vi "Send selected product.vi"(8 "error in (no error)":errorcluster, 10 "Product":i32, 11 "Coffee Actor in":refnum<class "Coffee Actor.lvclass">) -> (0 "error out":errorcluster, 3 "Coffee Actor out":refnum<class "Coffee Actor.lvclass">)   [LabVIEW 2020]
uses:
  <vilib>/ActorFramework/Actor/Actor.lvclass
  UI Actor Messages/Product Selected Msg/Product Selected Msg.lvclass
  Coffee Actor.lvclass
  C:/Program Files/National Instruments/LabVIEW 2020/vi.lib/ActorFramework/Actor/Actor.lvclass
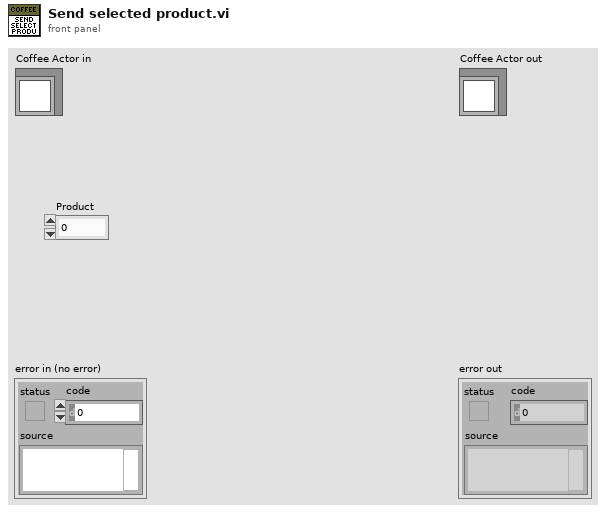
[diagram p1: front panel]
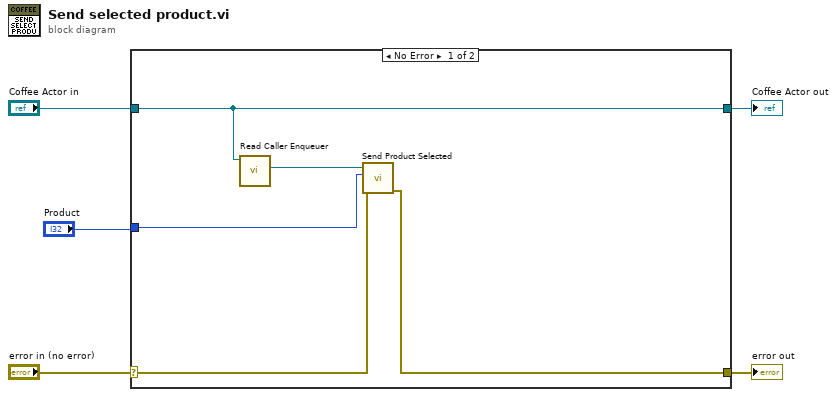
[diagram p0: block diagram]
diagram:
  n1 = case shown="No Error" "error in (no error)" {
    selector: "error in (no error)" -> [w7 w12]
    tunnel: [w6 w12] -> w4
    tunnel: [w10 w11] -> w2
    tunnel: "Coffee Actor in" -> [w10 w11]
    tunnel: "Product" -> [w8 _]
    frame No Error {
      n2 = call <vilib>:"Read Caller Enqueuer.vi"("Actor"=w10) -> ("Caller Enqueuer"=w9:refnum<class "Message Enqueuer.lvclass">)  [unwired: 10 in]
      n3 = call "Send Product Selected.vi"("error in (no error)"=w7, "Product Selected"=w8, "Message Enqueuer"=w9) -> ("error out"=w6:errorcluster)  [unwired: 7 in, 1 out]
    }
    frame Error {
    }
  }
  "error out" <- w4
  "Coffee Actor out" <- w2
